vi "Buy Actor.vi"(8 "error in (no error)":errorcluster, 10 "Producto":i32, 11 "coffe actor in":refnum<class "coffe actor.lvclass">) -> (0 "error out":errorcluster, 3 "coffe actor out":refnum<class "coffe actor.lvclass">)   [LabVIEW 2020, in "coffe actor.lvlib" / "coffe actor.lvclass"]
uses:
  coffe actor.lvclass
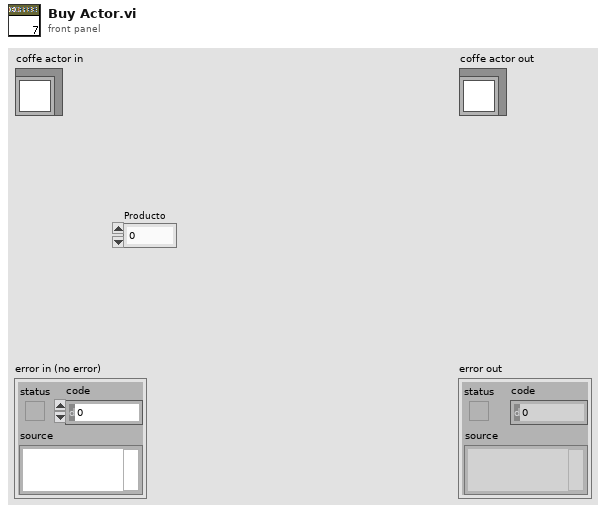
[diagram p1: front panel]
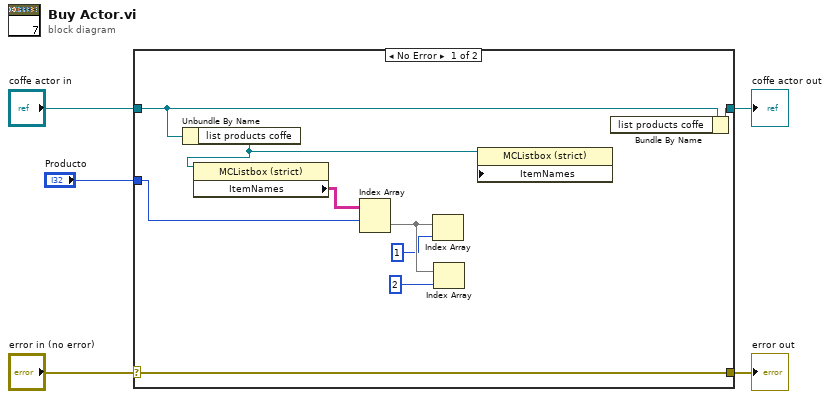
[diagram p0: block diagram]
diagram:
  n1 = case shown="No Error" "error in (no error)" {
    selector: "error in (no error)" -> [w14 w16]
    tunnel: [w14 w16] -> w4
    tunnel: [w7 w15] -> w2
    tunnel: "coffe actor in" -> [w8 w15]
    tunnel: "Producto" -> [w12 _]
    frame No Error {
      n2 = Unbundle By Name(w8) -> ("list products coffe"=w6:refnum<vi>)
      n3 = property class="MCListbox (strict)"(reference=w6) -> ("ItemNames"=w13:string[][])  [unwired: 1 in, 2 out]
      n4 = Index Array(array=w13, index (row)=w12) -> (element=w11:string[])  [unwired: 1 in]
      n5 = Index Array(array=w11, index=1) -> ()  [unwired: 1 out]
      n6 = Index Array(array=w11, index=2) -> ()  [unwired: 1 out]
      n7 = property class="MCListbox (strict)" props=["ItemNames"](reference=w6) -> ()  [unwired: 2 in, 2 out]
      n8 = Bundle By Name(cluster=w8) -> (w7:refnum<class "coffe actor.lvclass">)  [unwired: 1 in]
    }
    frame Error {
    }
  }
  "error out" <- w4
  "coffe actor out" <- w2
